vi "cv0.vi"() -> ()   [LabVIEW 2013]
panel:
  out "Numeric 2":dbl
  in  "Numeric":dbl
  out "Meter":u8(knob) scale=0.01..10.0
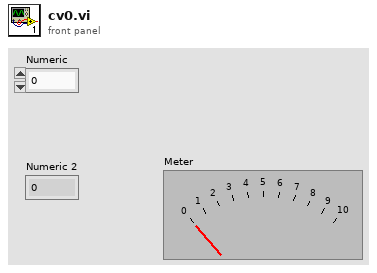
[diagram p1: front panel]
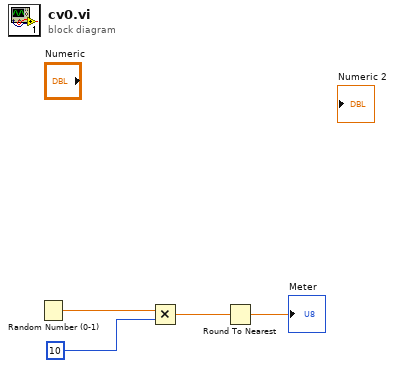
[diagram p0: block diagram]
diagram:
  n1 = Random Number (0-1)() -> (number: 0 to 1=w4:dbl)
  n2 = Multiply(x=w4, y=u32 10) -> (x*y=w2:dbl)
  n3 = Round To Nearest(number=w2) -> (nearest integer value=→"Meter":dbl)
